vi "VCS Move To Position.vi"(8 "error in (no error)":errorcluster, 9 "flags":cluster{"Absolute":i32, "Immediately":i32} {"Immediately" items=["false", "true"]; "Absolute" items=["false", "true"]}, 10 "targetPosition":i32, 11 "axis in":cluster{"keyHandle":u32, "nodeId":u16}={"keyHandle"=0, "nodeId"=1}) -> (0 "error out":errorcluster, 3 "axis out":cluster{"keyHandle":u32, "nodeId":u16}={"keyHandle"=0, "nodeId"=1})   [LabVIEW 2018]
doc: "With funciton <B>VCS Move To Position</B> device movement starts with position profile to target position."
uses:
  Resources/EposCmd.dll
  Resources/EposCmd64.dll
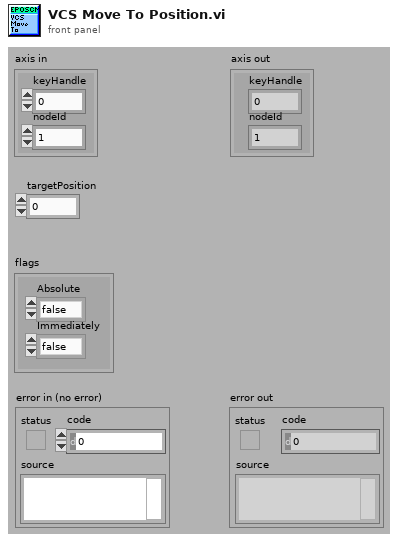
[diagram p1: front panel]
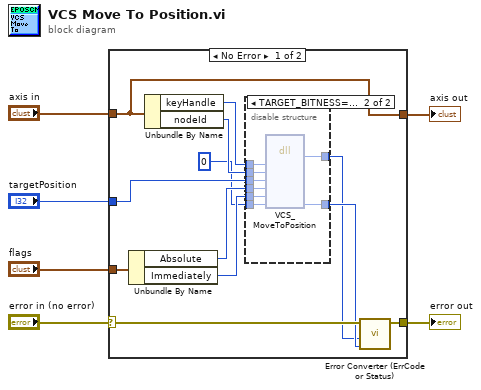
[diagram p0: block diagram]
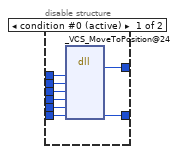
[diagram p2: hidden frame]
diagram:
  n1 = case shown="No Error" "error in (no error)" {
    selector: "error in (no error)" -> [w17 w36]
    tunnel: [w16 w36] -> w5
    tunnel: "targetPosition" -> [w18 _]
    tunnel: "flags" -> [w13 _]
    tunnel: "axis in" -> [w7 w35]
    tunnel: [w7 w35] -> w1
    frame No Error {
      n2 = Unbundle By Name(w13) -> ("Absolute"=w10:i32, "Immediately"=w9:i32)
      n3 = Unbundle By Name(w7) -> ("keyHandle"=w12:u32, "nodeId"=w11:u16)
      n4 = disable-structure shown="TARGET_BITNESS==64" {
        disable-tunnel: w18 -> [w26 w34]
        disable-tunnel: [w25 w33] -> w15
        disable-tunnel: [w24 w32] -> w14
        disable-tunnel: w12 -> [w23 w31]
        disable-tunnel: w11 -> [w22 w30]
        disable-tunnel: w10 -> [w21 w29]
        disable-tunnel: w9 -> [w20 w28]
        disable-tunnel: u32 0 ("pErrorCode") -> [w19 w27]
        frame condition #0 (active) {
          n5 = dll-call lib="C:/Projeto em LabVIEW/EPOS-LabVIEW-Instrument-Driver-En/LabVIEW/maxon EPOS/Resources/EposCmd.*" fn="_VCS_MoveToPosition@24"("KeyHandle"=w23, "NodeId"=w22, "TargetPosition"=w26, "Absolute"=w21, "Immediately"=w20, "pErrorCode"=w19) -> (w24:i32, "pErrorCode"=w25:u32)  [unwired: 8 in, 2 out]
        }
        frame condition #1 {
          n6 = dll-call lib="C:/setup/Resources/EposCmd64.*" fn="VCS_MoveToPosition" ("EposCmd.dll:_VCS_MoveToPosition@24")("KeyHandle"=w31, "NodeId"=w30, "TargetPosition"=w34, "Absolute"=w29, "Immediately"=w28, "pErrorCode"=w27) -> ("Rückgabetyp"=w32:i32, "pErrorCode"=w33:u32)  [unwired: 8 in, 2 out]
        }
      }
      n7 = call "Error Converter (ErrCode or Status).vi"("error code"=w15, "return type"=w14, "error in (no error)"=w17) -> ("error out"=w16:errorcluster)  [unwired: 7 in]
    }
    frame Error {
    }
  }
  "error out" <- w5
  "axis out" <- w1
